vi "Envira Main.vi"() -> ()   [LabVIEW 2023]
doc: "Use this template to build a simple state machine design pattern. Each state executes code and determines which state to transition to."
uses:
  Type Definitions/Envira State.ctl
  Type Definitions/Envira Data.ctl
panel:
  out "Read Data":string
  out "Start Read Loop":bool
  out "Stop Loop?":bool=TRUE
  out "Current Status":string
  in  "VISA resource name":refnum<visa-resource-name>
  in  "Turn PV OFF":bool
  in  "Turn PV ON":bool
  in  "Exit":bool
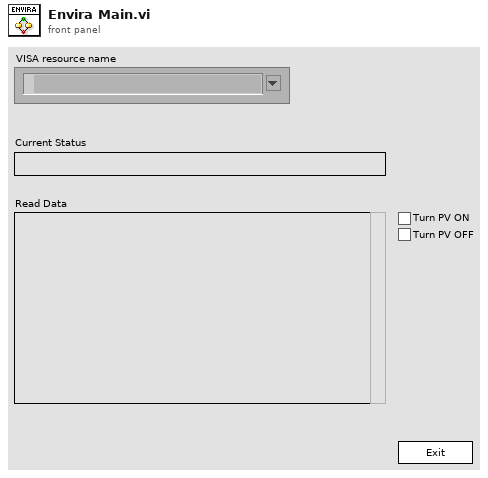
[diagram p1: front panel]
types:
  T1 = typedef "Envira Data.ctl" = cluster{"Current Status":string, "VISA resource name":refnum<visa-resource-name>, "Start Read Loop":bool}
  T2 = typedef "Envira State.ctl" = enum16{"Initialize", "Wait for Event", "Turn ON", "Turn OFF", "Exit"}
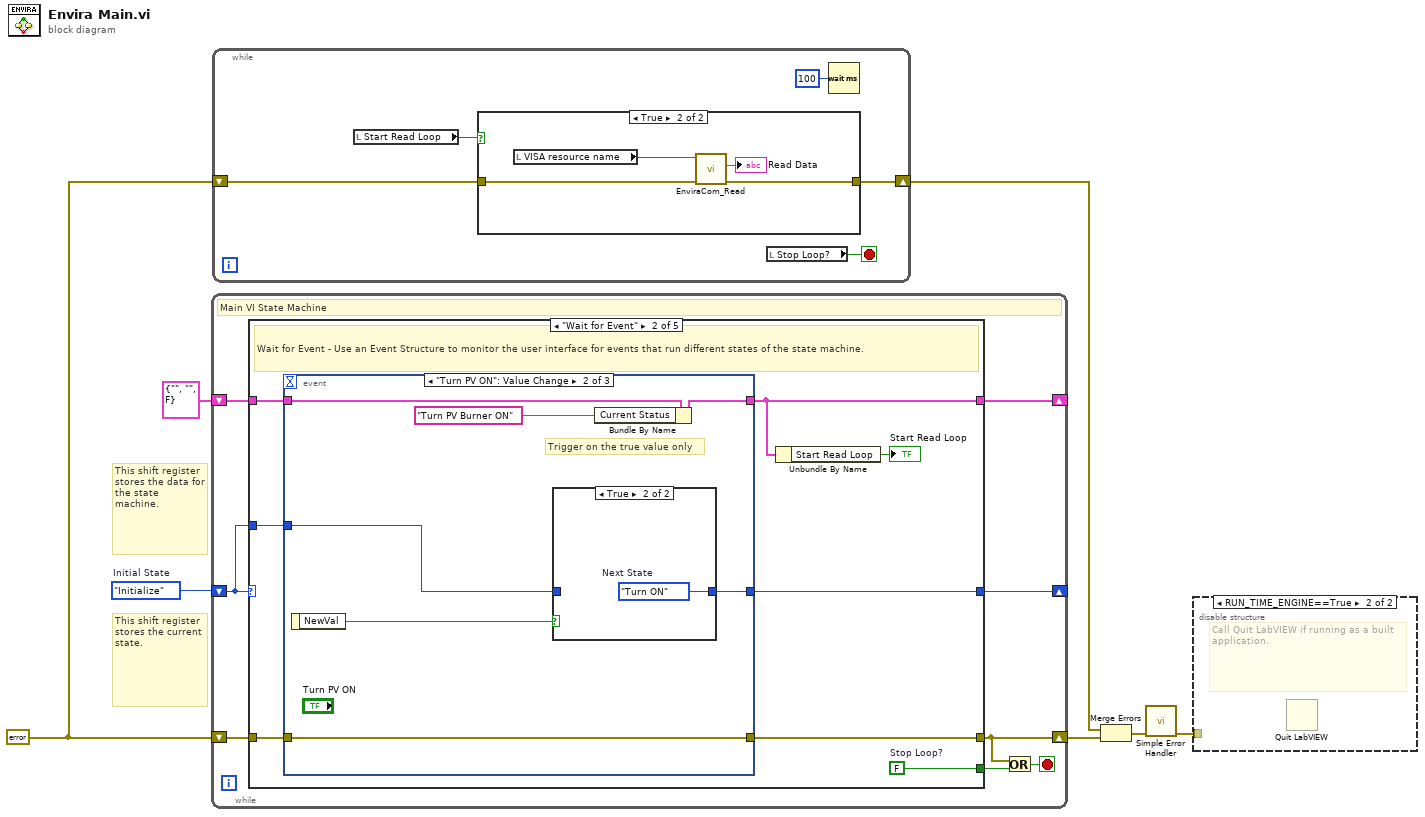
[diagram p0: block diagram]
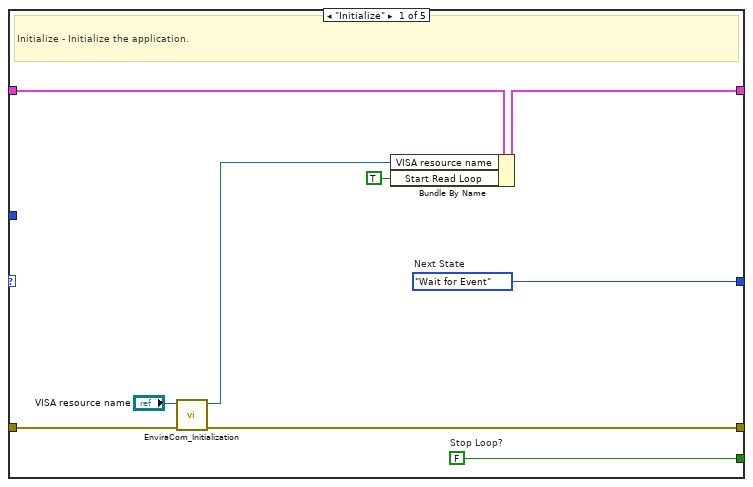
[diagram p4: hidden frame]
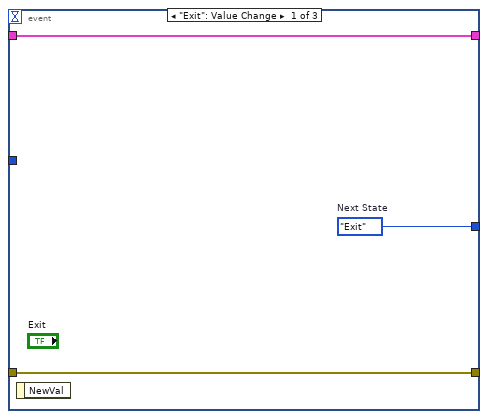
[diagram p5: hidden frame]
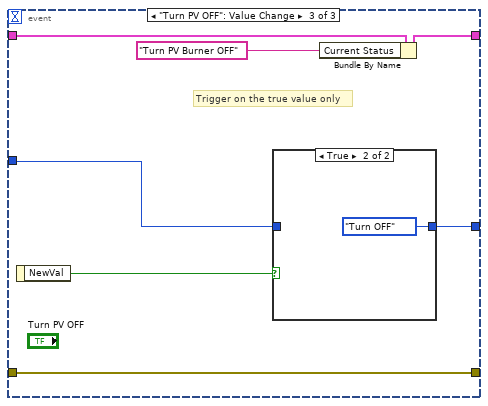
[diagram p7: hidden frame]
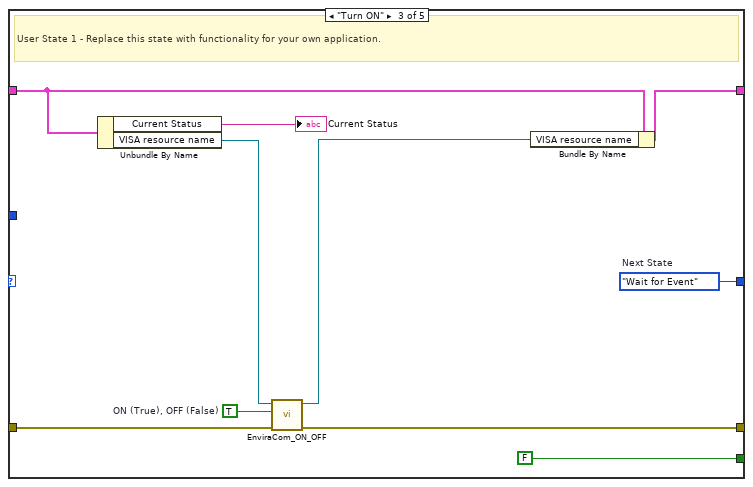
[diagram p9: hidden frame]
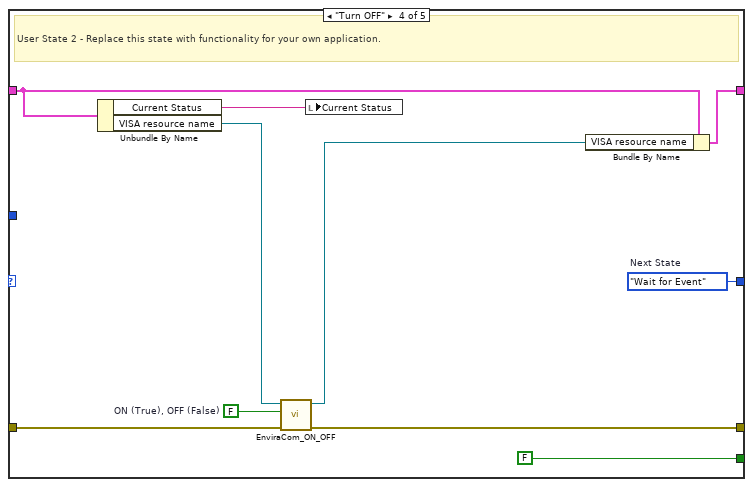
[diagram p10: hidden frame]
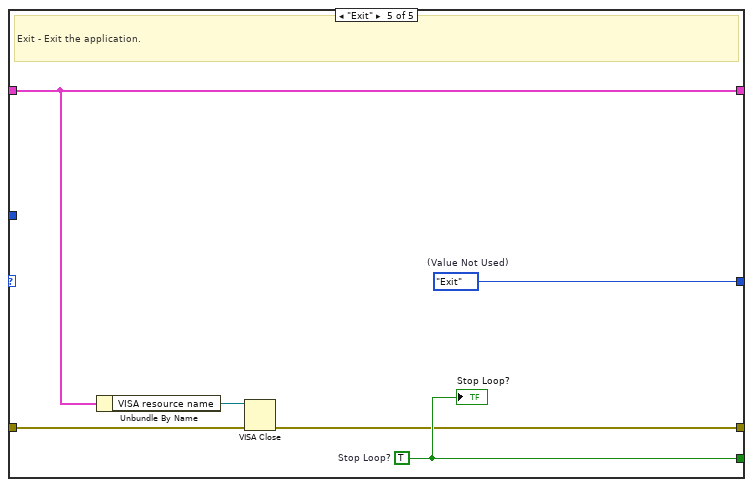
[diagram p11: hidden frame]
diagram:
  w4 = errorcluster {"status"=FALSE, "code"=0, "source"=""} ("error constant")
  w7 = Envira_State."Initialize"  # Initial State
  # "This shift register stores the data for the state machine."
  # "This shift register stores the current state."
  n1 = while {
    shift-right: [w15] -> _
    shift-left: w7 -> [w8]
    shift-right: [w13] -> _
    shift-left: T1 {"Current Status"="", "VISA resource name"="", "Start Read Loop"=FALSE} ("Data") -> [w14]
    shift-right: [w9] -> w2
    shift-left: w4 -> [w12]
    stop <- w10 stop-if-true
    # "Main VI State Machine"
    n2 = case shown="\"Wait for Event\"" w8 {
      tunnel: [w24 w32 w63 w73 w79] -> w15
      tunnel: [w23 w31 FALSE ("Stop Loop?") FALSE ("Stop Loop?") w78] -> w11
      tunnel: w14 -> [w22 w30 w56 w66 w77]
      tunnel: [w21 w27 w55 w65 w77] -> w13
      tunnel: w12 -> [w20 w29 w61 w70 w75]
      tunnel: [w19 w28 w60 w69 w74] -> w9
      tunnel: w8 -> [_ w25 _ _ _]
      frame "Initialize" {
        w23 = FALSE  # Stop Loop?
        w24 = Envira_State."Wait for Event"  # Next State
        # "Initialize - Initialize the application."
        n3 = call "EnviraCom_Initialization.vi"("error in (no error)"=w20, "VISA Refnum in"="VISA resource name") -> ("error out"=w19:errorcluster, "VISA Refnum out"=w17:refnum<visa-resource-name>)  [unwired: 8 in]
        n4 = Bundle By Name(cluster=w22, "VISA resource name"=w17, "Start Read Loop"=TRUE) -> (w21:T1)
      }
      frame "Wait for Event" {
        w31 = FALSE  # Stop Loop?
        # "Wait for Event - Use an Event Structure to monitor the user interface for events that run different states of the state machine."
        n5 = event shown="[1] \"Turn PV ON\": Value Change" {
          selector: _ -> [_ _ _]
          dyn-events: _ -> [_ _ _]
          timeout: _ -> [_ _ _]
          tunnel: [w35 w42 w51] -> w32
          tunnel: w30 -> [w34 w41 w50]
          tunnel: [w34 w40 w49] -> w27
          tunnel: w29 -> [w33 w38 w47]
          tunnel: [w33 w38 w47] -> w28
          tunnel: w25 -> [_ w36 w45]
          event "Exit": Value Change {
            w35 = Envira_State."Exit"  # Next State
            n6 = event-data() -> ()  [unwired: 1 in, 1 out]
          }
          event "Turn PV ON": Value Change {
            # "Trigger on the true value only"
            n7 = event-data() -> ("NewVal"=w37:bool)  [unwired: 1 in]
            n8 = case shown="True" w37 {
              tunnel: [w43 w44] -> w42
              tunnel: w36 -> [w43 _]
              frame False {
              }
              frame True {
                w44 = Envira_State."Turn ON"  # Next State
              }
            }
            n9 = Bundle By Name(cluster=w41, "Current Status"="Turn PV Burner ON" ("Running User State 1")) -> (w40:T1)
          }
          event "Turn PV OFF": Value Change {
            # "Trigger on the true value only"
            n10 = event-data() -> ("NewVal"=w46:bool)  [unwired: 1 in]
            n11 = case shown="True" w46 {
              tunnel: [w52 Envira_State."Turn OFF" ("Next State")] -> w51
              tunnel: w45 -> [w52 _]
              frame False {
              }
              frame True {
              }
            }
            n12 = Bundle By Name(cluster=w50, "Current Status"="Turn PV Burner OFF" ("Running User State 2")) -> (w49:T1)
          }
        }
        n13 = Unbundle By Name(w27) -> ("Start Read Loop"=→"Start Read Loop":bool)
      }
      frame "Turn ON" {
        w57 = TRUE  # ON (True), OFF (False)
        w63 = Envira_State."Wait for Event"  # Next State
        # "User State 1 - Replace this state with functionality for your own application."
        n14 = Unbundle By Name(w56) -> ("Current Status"=→"Current Status":string, "VISA resource name"=w58:refnum<visa-resource-name>)
        n15 = call "EnviraCom_ON_OFF.vi"("error in (no error)"=w61, "ON (True), OFF (False)"=w57, "VISA Refnum in"=w58) -> ("error out"=w60:errorcluster, "VISA Refnum out"=w54:refnum<visa-resource-name>)  [unwired: 7 in]
        n16 = Bundle By Name(cluster=w56, "VISA resource name"=w54) -> (w55:T1)
      }
      frame "Turn OFF" {
        w67 = FALSE  # ON (True), OFF (False)
        w73 = Envira_State."Wait for Event"  # Next State
        # "User State 2 - Replace this state with functionality for your own application."
        n17 = Unbundle By Name(w66) -> ("Current Status"=w71:string, "VISA resource name"=w68:refnum<visa-resource-name>)
        n18 = call "EnviraCom_ON_OFF.vi"("error in (no error)"=w70, "ON (True), OFF (False)"=w67, "VISA Refnum in"=w68) -> ("error out"=w69:errorcluster, "VISA Refnum out"=w64:refnum<visa-resource-name>)  [unwired: 7 in]
        n19 = local write "Current Status"(w71) -> ()
        n20 = Bundle By Name(cluster=w66, "VISA resource name"=w64) -> (w65:T1)
      }
      frame "Exit" {
        w78 = TRUE  # Stop Loop?
        w79 = Envira_State."Exit"  # (Value Not Used)
        # "Exit - Exit the application."
        n21 = Unbundle By Name(w77) -> ("VISA resource name"=w76:refnum<visa-resource-name>)
        n22 = VISA Close(VISA resource name=w76, error in (no error)=w75) -> (error out=w74:errorcluster)
        "Stop Loop?" <- w78
      }
    }
    n23 = Or(x=w9, y=w11) -> (x .or. y?=w10:bool)
  }
  n24 = while {
    shift-right: [w81] -> w3
    shift-left: w4 -> [w82]
    stop <- w84 stop-if-true
    n25 = local read "Start Read Loop"() -> (w80:bool)
    n26 = case shown="True" w80 {
      tunnel: w82 -> [w85 w88]
      tunnel: [w85 w87] -> w81
      frame False {
      }
      frame True {
        n27 = local read "VISA resource name"() -> (w89:refnum<visa-resource-name>)
        n28 = call "EnviraCom_Read.vi"("error in (no error)"=w88, "VISA Refnum in"=w89) -> ("error out"=w87:errorcluster, "Read Data"=→"Read Data":string)  [unwired: 7 in, 1 out]
      }
    }
    n29 = local read "Stop Loop?"() -> (w84:bool)
    n30 = Wait (ms)(milliseconds to wait=u32 100) -> ()  [unwired: 1 out]
  }
  n31 = Merge Errors(w3, w2) -> (w1:errorcluster)
  n32 = call <vilib>:"Simple Error Handler.vi"("error in (no error)"=w1) -> ("error out"=w5:errorcluster)  [unwired: 4 in, 4 out]
  n33 = disable-structure shown="RUN_TIME_ENGINE==True" {
    disable-tunnel: w5 -> [_ _]
    frame condition #0 (active) {
    }
    frame condition #1 {
      # "Call Quit LabVIEW if running as a built application."
      n34 = Quit LabVIEW() -> ()  [unwired: 1 in]
    }
  }
